vi "AutoTurnSubVi.vi"(4 "I":dbl, 5 "Speed":dbl, 6 "P":dbl, 7 "D":dbl, 8 "navX Device":T1 {"Interface"."Update Rate (4Hz-60Hz)" min=4 max=60 step=1}, 9 "Angle":dbl, 10 "VDeadband":dbl, 11 "Deadband":dbl) -> (2 "Output":dbl format="%#_13g", 3 "Boolean":bool)   [LabVIEW 2016]
uses:
  NavX/navX Library v2/TypeDefs/Z900_navX_DeviceTypeDef.ctl
  NavX/navX Library v2/TypeDefs/Z900_navX_ProtocolTypeDef.ctl
  NavX/navX Library v2/TypeDefs/Z900_navX_NotifyPacketTypeDef.ctl
  NavX/navX Library v2/TypeDefs/Z900_navX_ActionTypeDef.ctl
  <vilib>/Rock Robotics/Network Tables/NT Write Boolean.vi
  <vilib>/Rock Robotics/Network Tables/NT Write Number.vi
  <vilib>/addons/control/pid/pid.llb/PID (DBL).vi
  <vilib>/addons/control/pid/NI_PID_pid.lvlib
  NavX/navX Library v2/navX Library v2.lvlib
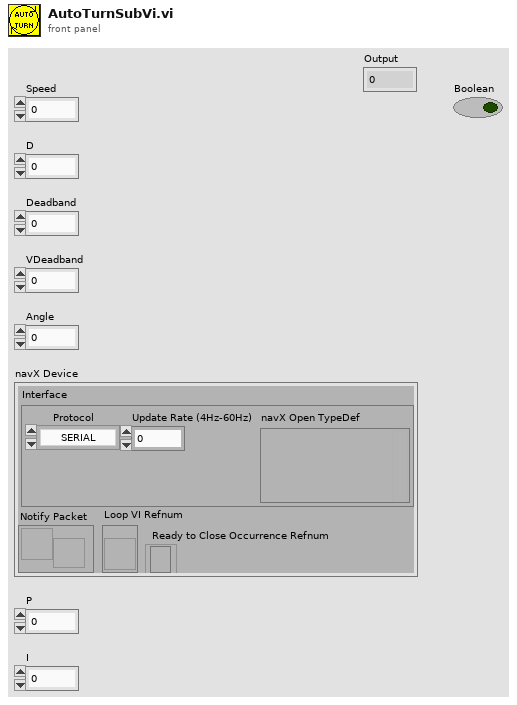
[diagram p1: front panel]
types:
  T1 = typedef "navX Library v2.lvlib/Z900_navX_DeviceTypeDef.ctl" = cluster{"Interface":cluster{"Protocol":T2, "Update Rate (4Hz-60Hz)":u8, "navX Open TypeDef":variant}, "Notify Packet":refnum<notifier>, "Loop VI Refnum":refnum<vi>, "Ready to Close Occurrence Refnum":refnum<k4>}
  T2 = typedef "navX Library v2.lvlib/Z900_navX_ProtocolTypeDef.ctl" = enum16{"SERIAL", "I2C", "SPI"}
  T3 = cluster{"Accel X":dbl, "Accel Y":dbl, "Accel Z":dbl, "Gyro X":dbl, "Gyro Y":dbl, "Gyro Z":dbl, "Mag X":dbl, "Mag Y":dbl, "Mag Z":dbl}
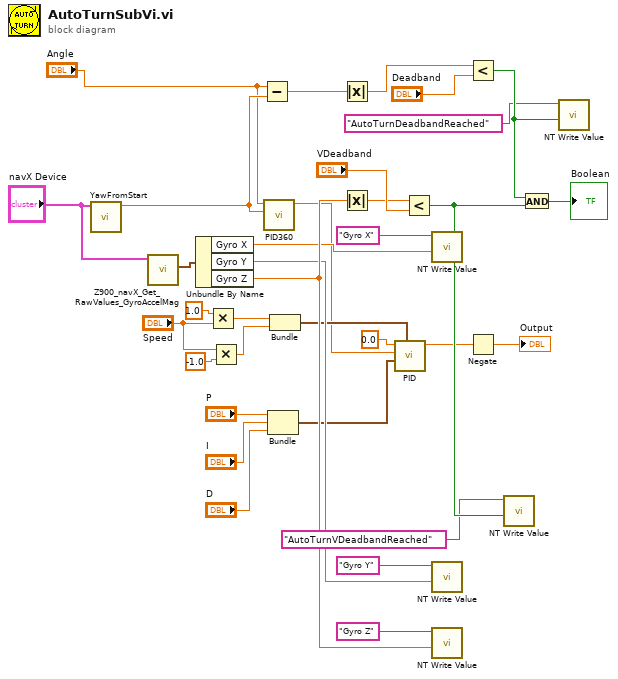
[diagram p0: block diagram]
diagram:
  n1 = call "YawFromStart.vi"("navX Device"="navX Device") -> ("Yaw"=w15:dbl)  [unwired: 10 in]
  n2 = call "Z900_navX_Get_RawValues_GyroAccelMag.vi"("navX Device"="navX Device") -> ("Raw Values"=w17:T3)  [unwired: 7 in, 3 out]
  n3 = Unbundle By Name(w17) -> ("Gyro X"=w18:dbl, "Gyro Y"=w19:dbl, "Gyro Z"=w23:dbl)
  n4 = Multiply(x=1.0, y="Speed") -> (x*y=w8:dbl)
  n5 = Multiply(x="Speed", y=-1.0) -> (x*y=w7:dbl)
  n6 = Subtract(x="Angle", y=w15) -> (x-y=w12:dbl)
  n7 = call "PID360.vi"("Robot"=w15, "Target"="Angle") -> ("Numeric"=w2:dbl)  [unwired: 9 in]
  n8 = Bundle("P"="P", "I"="I", "D"="D") -> (w10:cluster{"P":dbl, "I":dbl, "D":dbl})  [unwired: 1 in]
  n9 = Bundle(w8, w7) -> (w9:cluster{dbl, dbl})  [unwired: 1 in]
  n10 = Absolute Value(x=w12) -> (abs(x)=w13:dbl)
  n11 = Absolute Value(x=w23) -> (abs(x)=w24:dbl)
  n12 = call-poly <vilib>:"PID.vi"("output range"=w9, "PID gains"=w10, "process variable"=w2, "setpoint"=0.0) -> ("output"=w11:dbl)  [unwired: 6 in, 1 out]
  n13 = Less?(x=w24, y="VDeadband") -> (x < y?=w28:bool)
  n14 = call-poly <vilib>:"NT Write Value.vi"("Numeric"=w18, "Name"="Gyro X") -> ()  [unwired: 9 in, 1 out]
  n15 = call-poly <vilib>:"NT Write Value.vi"("Numeric"=w19, "Name"="Gyro Y") -> ()  [unwired: 9 in, 1 out]
  n16 = call-poly <vilib>:"NT Write Value.vi"("Numeric"=w23, "Name"="Gyro Z") -> ()  [unwired: 9 in, 1 out]
  n17 = Less?(x=w13, y="Deadband") -> (x < y?=w29:bool)
  n18 = Negate(x=w11) -> (-x=→"Output":dbl)
  n19 = call-poly <vilib>:"NT Write Value.vi"("Boolean"=w28, "Name"="AutoTurnVDeadbandReached") -> ()  [unwired: 9 in, 1 out]
  n20 = And(x=w29, y=w28) -> (x .and. y?=→"Boolean":bool)
  n21 = call-poly <vilib>:"NT Write Value.vi"("Boolean"=w29, "Name"="AutoTurnDeadbandReached") -> ()  [unwired: 9 in, 1 out]
